vi "Z-Scan-Simulation-Analysis-first-point.vi"() -> ()   [LabVIEW 2014]
doc: "André Romero - 2016\nandretec@ifsc.usp.br"
uses:
  <vilib>/Analysis/baseanly.llb/Mean (DBL).vi
  <vilib>/Utility/file.llb/Write To Spreadsheet File (DBL).vi
  <vilib>/Analysis/NI_AALBase.lvlib
panel:
  out "error (%)":dbl(graph)
  out "Waveform Graph":dbl[][](graph)
  out "Delay VI mean":dbl=63.55555555555556 format="%0.2f"
  out "Delay DAQ mean":dbl=253.55555555555554 format="%0.2f"
  in  "stop":bool
  out "Process time":string="0:00:27"
  out "Array":dbl[](array[numeric])=[2.7399115920461927]
  out "delay (ms)":u32=27328
  in  "milliseconds to wait":u32
  out "mean tf/ti":dbl=2.7399115920461927 format="%0.3f"
  out "status media":i32
  in  "Médias":i32=1 min=1
  out "min value":dbl=2.716291312943804
  out "max value":dbl=2.7530073421259127
  out "Dellay VI":u32(graph)=9
  out "Delay DAQ":u32(graph)=252
  in  "number of samples":i32=40000
  in  "rate":dbl=200000.0 format="%#_13g"
  out "variance":dbl=4.33248215247306e-05 format="%0.6f"
  out "standard deviation":dbl=0.006582159336018128 format="%0.6f"
  out "mean":dbl=2.736901171579517 format="%0.6f"
  out "Delta voltage":dbl=0.03671602918210848 format="%#_8g"
  out "Number of samples":i32=9
  in  "Save ?":bool=TRUE
  in  "delay between points (ms)":u32
  out "Z-Scan Graph":dbl[](graph)=[2.735132708454353, 2.738947350836858, 2.734655244051734, 2.7396822438623687, 2.7278277474129107, 2.7387763962228693, 2.736558085660297, 2.7323997631539765, 2.738221107624196, 2.7393305632862397, 2.741314993759599, 2.747504778022689, 2.738857646673517, 2.730907003892475, 2.732997610548393, 2.7267654500428216, 2.7348215281721826, 2.737937468343614, 2.726070168151901, 2.731887449619976, 2.732414299906183, 2.7330931378202687, 2.716291312943804, 2.7303619340530645, 2.7369114862989874, 2.731523112752885, 2.7354675161048174, 2.7298018305712075, 2.7284991278572837, 2.737353103281323, 2.7327358431598725, 2.734910344261488, 2.7378594937125103, 2.7502146828530214, 2.7337306242369928, 2.739842480175337, 2.7315173269319546, 2.738028284846607, 2.75184747183654, 2.734010133292254, 2.739883879966676, 2.7530073421259127, 2.7364398773661778, 2.7380245402985475, 2.746210731914264, 2.74784258473236, 2.746055600985261, 2.744685689686615, 2.7373947781805184, 2.742865724075715, 2.7398119555480935, 2.7460854422451066, 2.741835143466216, 2.724498522334739, 2.7360680289422383, 2.7324008327222256, 2.7296285024348417, 2.733434961351708, 2.741336308672092, 2.7279657751965862, 2.740709507192904, 2.7400586240991918, 2.739035501835608, 2.7442928765615813, 2.736082802692787, 2.7289248052339135, 2.734834467568928, 2.7227483022204564, 2.73278233554788, 2.732269078647335, 2.7273725581509534, 2.7374985614049385, 2.7403197210099997, 2.7428918309602253, 2.7494572970150637, 2.7288847122884303, 2.7411122138760424, 2.7408703110680195, 2.7347213443213247, 2.7386168772101653, 2.7320536866131246, 2.7323118031594973, 2.7421055815034725, 2.741757853433335, 2.732606885118174, 2.7258367239769905, 2.7501519595100596, 2.737371798824078, 2.731794368257389, 2.7411112883575326, 2.7319720404070353, 2.7423628600299246, 2.7386655586714026, 2.738447831787006, 2.744117336184531, 2.740055256798649, 2.7381788823262183, 2.7463663278142176, 2.7369687172918487, 2.7399115920461927]
  in  "N Points":i32=100
  in  "GO":bool
  out "Z-Scan graph":dbl[][](graph)
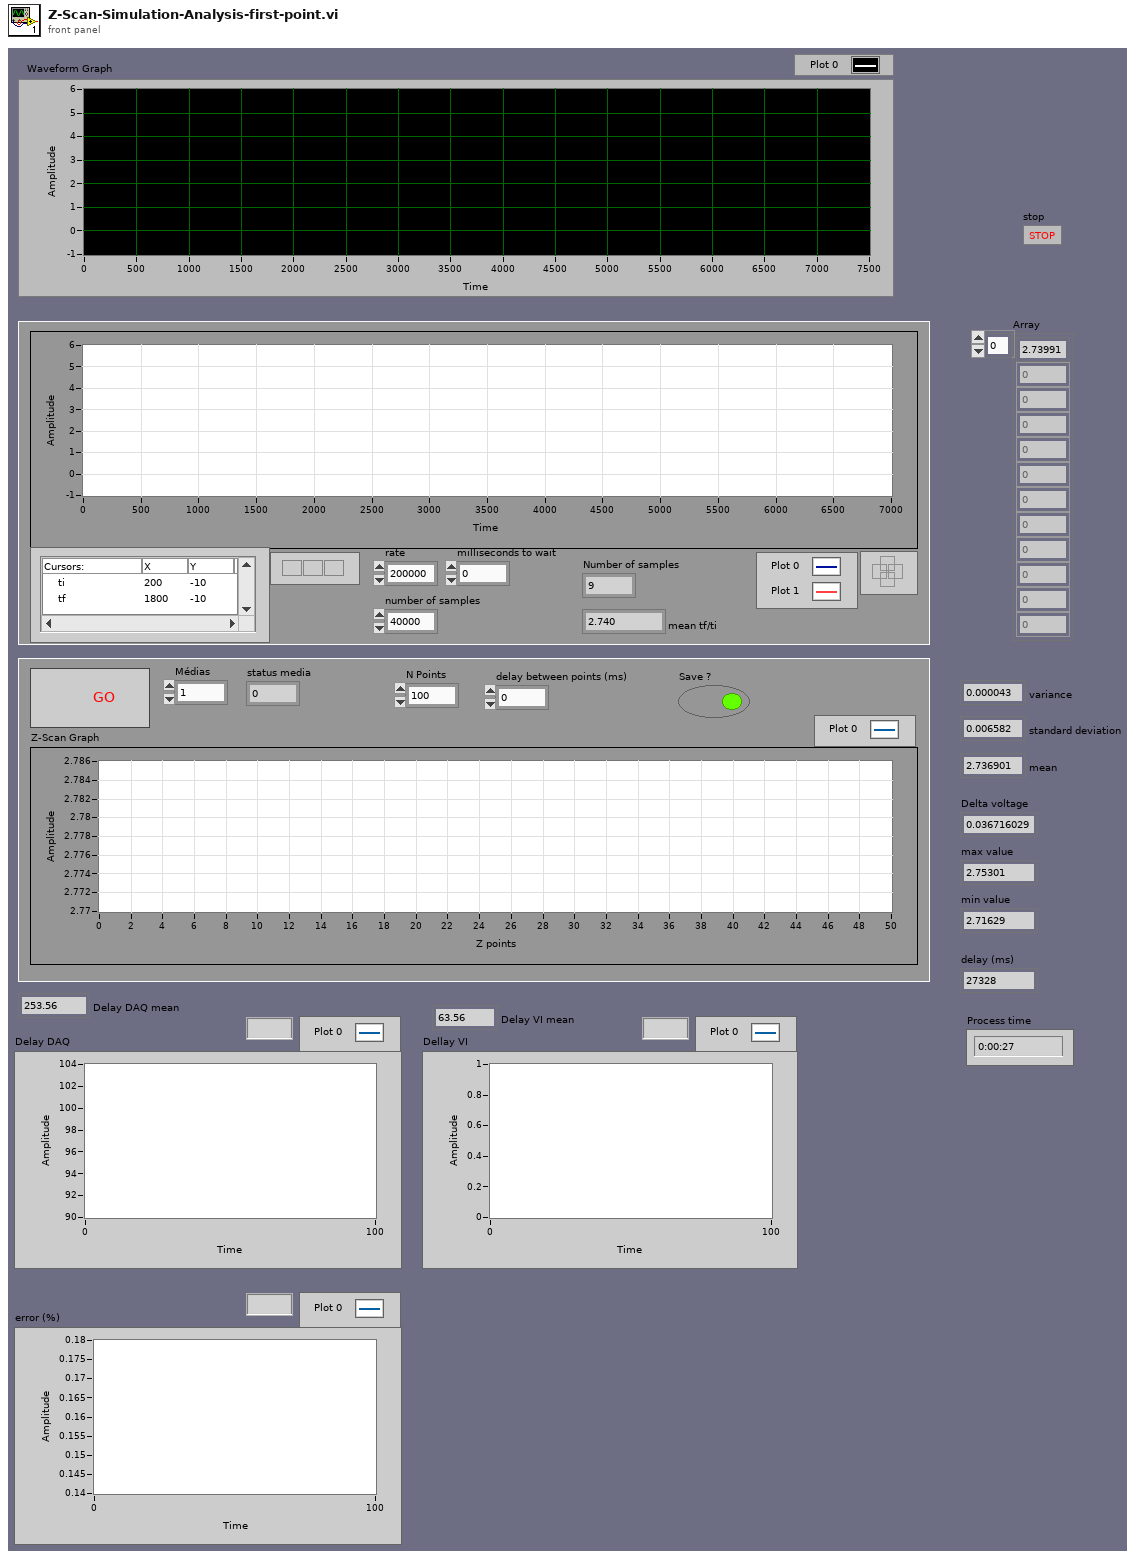
[diagram p1: front panel]
types:
  T1 = typedef "LVCursorListTypeDef.ctl" = cluster{"Name":string, "Color":u32, "Style":u8, "Point Style":u8, "Name Visible":bool, "Allow Drag":bool, "Cursor Mode":u32, "Plot":i32, "Index":i32, "Position":cluster{"X":dbl, "Y":dbl}, "X Scale":u32, "Y Scale":u32, "Watch Plots":i32[], "Watch All Plots":bool, "Plot Area":i32, "Label Offset":cluster{"X":dbl, "Y":dbl}}[]
  T2 = cluster{"Name":string, "Color":u32, "Style":u8, "Point Style":u8, "Name Visible":bool, "Allow Drag":bool, "Cursor Mode":u32, "Plot":i32, "Index":i32, "Position":cluster{"X":dbl, "Y":dbl}, "X Scale":u32, "Y Scale":u32, "Watch Plots":i32[], "Watch All Plots":bool, "Plot Area":i32, "Label Offset":cluster{"X":dbl, "Y":dbl}}
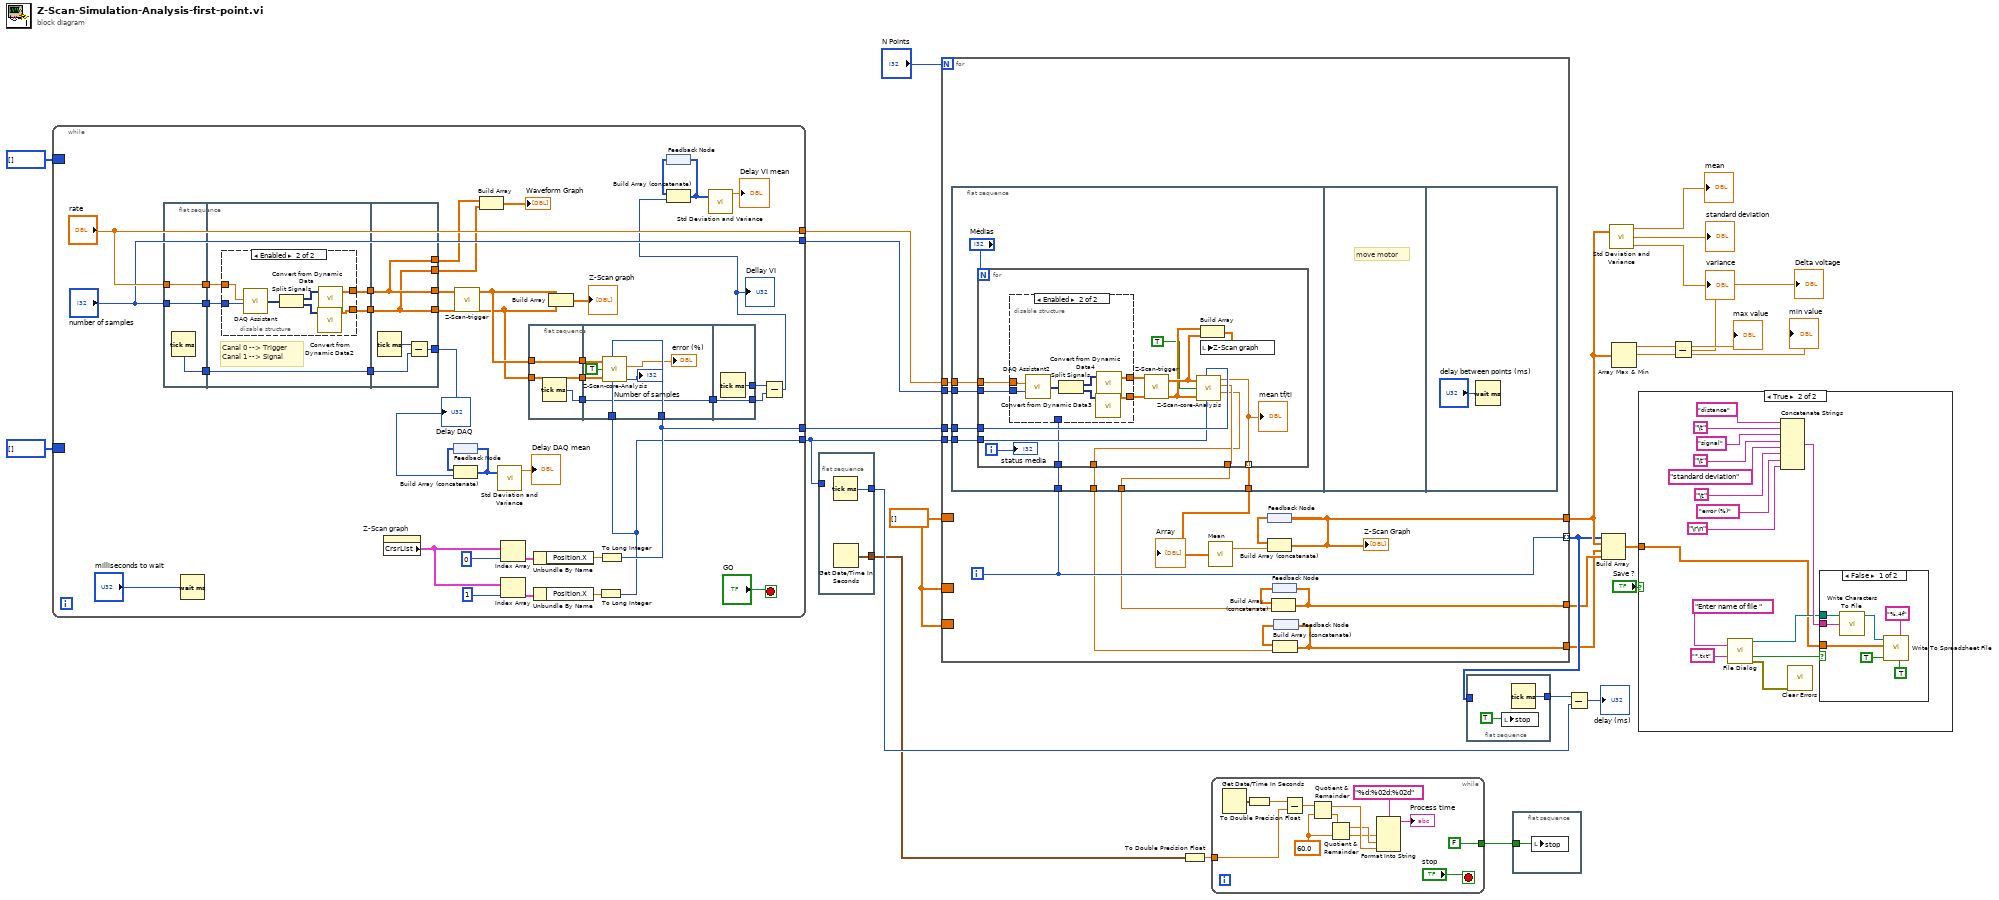
[diagram p0: block diagram]
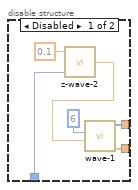
[diagram p2: hidden frame]
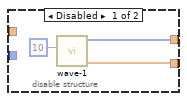
[diagram p3: hidden frame]
diagram:
  w3 = dbl[] []
  n1 = while {
    tunnel: [w58] -> w26
    tunnel: [w57] -> w13
    tunnel: ["rate"] -> w22
    tunnel: ["number of samples"] -> w21
    border: u32[] [] -> [_]
    border: u32[] [] -> [_]
    stop <- "GO" stop-if-true
    n2 = flat-sequence {
      tunnel: "number of samples" -> [w82]
      tunnel: "rate" -> [w83]
      tunnel: [w83] -> w51
      tunnel: [w82] -> w50
      tunnel: [w81] -> w47
      tunnel: w51 -> [w86]
      tunnel: w50 -> [w85]
      tunnel: [w88] -> w49
      tunnel: [w87] -> w48
      tunnel: w47 -> [w84]
      tunnel: [w84] -> w46
      tunnel: [w99] -> w55
      tunnel: [w100] -> w56
      tunnel: w49 -> [w100]
      tunnel: w48 -> [w99]
      tunnel: w46 -> [w102]
      tunnel: [w101] -> w37
      tunnel: [w100] -> w29
      tunnel: [w99] -> w28
      frame #0 {
        n3 = Tick Count (ms)() -> (millisecond timer value=w81:u32)
      }
      frame #1 {
        # "Canal 0 --> Trigger\nCanal 1 --> Signal"
        n4 = disable-structure shown="Enabled" {
          disable-tunnel: [w90 w95] -> w88
          disable-tunnel: [w89 w94] -> w87
          disable-tunnel: w86 -> [_ w98]
          disable-tunnel: w85 -> [_ w97]
          frame Disabled {
            n5 = call "wave-1.vi"("N cycles"=i64 10) -> ("signal"=w89:dbl[], "trigger"=w90:i32[])  [unwired: 7 in]
          }
          frame Enabled {
            n6 = call "DAQ Assistant"("rate"=w98, "number of samples"=w97) -> ("data"=w96:dynamicdata)  [unwired: 15 in, 2 out]
            n7 = Split Signals(w96) -> (w92:dynamicdata, w93:dynamicdata)  [unwired: 2 in]
            n8 = call "Convert from Dynamic Data2"("Dynamic Data Type"=w93) -> ("Array"=w94:dbl[])  [unwired: 3 in]
            n9 = call "Convert from Dynamic Data"("Dynamic Data Type"=w92) -> ("Array"=w95:dbl[])  [unwired: 3 in]
          }
        }
      }
      frame #2 {
        n10 = Tick Count (ms)() -> (millisecond timer value=w103:u32)
        n11 = Subtract(x=w103, y=w102) -> (x-y=w101:u32)
      }
    }
    n12 = Wait (ms)(milliseconds to wait="milliseconds to wait") -> ()  [unwired: 1 out]
    n13 = property on="Z-Scan graph" class="WFGraph (strict)"() -> ("CrsrList"=w66:T1)  [unwired: 2 in, 2 out]
    n14 = feedback #1() -> (w38:u32[])
    n15 = Build Array (concatenate)(w38, w37) -> (w36:u32[])
    n16 = feedback-in #1(w36) -> ()
    n17 = call "Z-Scan-trigger.vi"("signal in"=w55, "trigger in"=w56) -> ("signal out"=w30:dbl[], "trigger out"=w54:dbl[])  [unwired: 5 in, 1 out]
    n18 = Build Array(w29, w28) -> (→"Waveform Graph":dbl[][])
    n19 = call <vilib>:"Std Deviation and Variance.vi"("X"=w36) -> ("mean"=→"Delay DAQ mean":dbl)  [unwired: 1 in, 2 out]
    n20 = Index Array(array=w66, index=0) -> (element=w64:T2)
    n21 = Index Array(array=w66, index=1) -> (element=w63:T2)
    n22 = flat-sequence {
      tunnel: w30 -> [w69]
      tunnel: w54 -> [w70]
      tunnel: [w70] -> w45
      tunnel: [w69] -> w44
      tunnel: [w68] -> w42
      tunnel: w58 -> [w77]
      tunnel: w57 -> [w76]
      tunnel: w45 -> [w75]
      tunnel: w44 -> [w74]
      tunnel: w42 -> [w73]
      tunnel: [w73] -> w41
      tunnel: [w80] -> w43
      tunnel: w41 -> [w79]
      tunnel: [w79] -> w40
      frame #0 {
        n23 = Tick Count (ms)() -> (millisecond timer value=w68:u32)
      }
      frame #1 {
        n24 = call "Z-Scan-core-Analysis.vi"("trigger in"=w75, "ti"=w77, "First point"=TRUE, "signal in"=w74, "tf"=w76) -> ("error (%)"=→"error (%)":dbl, "number of samples"=→"Number of samples":i32)  [unwired: 2 out]
      }
      frame #2 {
        n25 = Tick Count (ms)() -> (millisecond timer value=w80:u32)
      }
    }
    n26 = Unbundle By Name(w64) -> ("Position.X"=w62:dbl)
    n27 = Unbundle By Name(w63) -> ("Position.X"=w61:dbl)
    n28 = Build Array(w30, w54) -> (→"Z-Scan graph":dbl[][])
    n29 = To Long Integer(number=w61) -> (32bit integer=w57:i32)
    n30 = To Long Integer(number=w62) -> (32bit integer=w58:i32)
    n31 = feedback #2() -> (w34:u32[])
    n32 = Subtract(x=w43, y=w40) -> (x-y=w33:u32)
    "Dellay VI" <- w33
    n33 = Build Array (concatenate)(w34, w33) -> (w32:u32[])
    n34 = feedback-in #2(w32) -> ()
    n35 = call <vilib>:"Std Deviation and Variance.vi"("X"=w32) -> ("mean"=→"Delay VI mean":dbl)  [unwired: 1 in, 2 out]
    "Delay DAQ" <- w37
  }
  n36 = flat-sequence {
    tunnel: w13 -> [_]
    tunnel: [w105] -> w10
    tunnel: [w104] -> w7
    frame #0 {
      n37 = Tick Count (ms)() -> (millisecond timer value=w105:u32)
      n38 = Get Date/Time In Seconds() -> (seconds since 1Jan1904=w104:timestamp)
    }
  }
  n39 = for {
    N: "N Points" -> [_]
    tunnel: w26 -> [w120]
    tunnel: w13 -> [w119]
    tunnel: [w117] -> w12 mode=indexing
    border: w3 -> [_]
    tunnel: [w116] -> w14
    tunnel: w22 -> [w115]
    tunnel: w21 -> [w114]
    border: w3 -> [_]
    tunnel: [w109] -> w2
    border: w3 -> [_]
    tunnel: [w106] -> w1
    i -> [w117]
    n40 = flat-sequence {
      tunnel: w120 -> [w129]
      tunnel: w119 -> [w128]
      tunnel: [w127] -> w113
      tunnel: w117 -> [w126]
      tunnel: w115 -> [w125]
      tunnel: w114 -> [w124]
      tunnel: [w122] -> w110
      tunnel: [w121] -> w107
      frame #0 {
        n41 = for {
          N: "Médias" -> [_]
          tunnel: w129 -> [w144]
          tunnel: w128 -> [w143]
          tunnel: [w142] -> w127 mode=indexing
          tunnel: w126 -> [w136]
          tunnel: w125 -> [w135]
          tunnel: w124 -> [w134]
          tunnel: [w131] -> w122
          tunnel: [w130] -> w121
          i -> [w133]
          n42 = disable-structure shown="Enabled" {
            disable-tunnel: [w150 w154] -> w141
            disable-tunnel: [w149 w153] -> w140
            disable-tunnel: w136 -> [w145 _]
            disable-tunnel: w135 -> [_ w152]
            disable-tunnel: w134 -> [_ w151]
            frame Disabled {
              n43 = call "z-wave-2.vi"("index"=w145, "amplitutude"=0.1) -> ("element"=w146:dbl)  [unwired: 1 in, 2 out]
              n44 = call "wave-1.vi"("slope"=w146, "N cycles"=i64 6) -> ("signal"=w149:dbl[], "trigger"=w150:i32[])  [unwired: 6 in]
            }
            frame Enabled {
              n45 = call "DAQ Assistant2"("rate"=w152, "number of samples"=w151) -> ("data"=w155:dynamicdata)  [unwired: 15 in, 2 out]
              n46 = Split Signals(w155) -> (w157:dynamicdata, w156:dynamicdata)  [unwired: 2 in]
              n47 = call "Convert from Dynamic Data3"("Dynamic Data Type"=w156) -> ("Array"=w153:dbl[])  [unwired: 3 in]
              n48 = call "Convert from Dynamic Data4"("Dynamic Data Type"=w157) -> ("Array"=w154:dbl[])  [unwired: 3 in]
            }
          }
          n49 = call "Z-Scan-trigger.vi"("signal in"=w140, "trigger in"=w141) -> ("signal out"=w137:dbl[], "trigger out"=w138:dbl[])  [unwired: 5 in, 1 out]
          n50 = call "Z-Scan-core-Analysis.vi"("trigger in"=w138, "ti"=w144, "First point"=TRUE, "signal in"=w137, "tf"=w143) -> ("mean tf/ti"=w142:dbl, "error (%)"=w131:dbl, "standard deviation"=w130:dbl)  [unwired: 1 out]
          "mean tf/ti" <- w142
          n51 = Build Array(w137, w138) -> (w139:dbl[][])
          n52 = local write "Z-Scan graph"(w139) -> ()
          "status media" <- w133
        }
      }
      frame #1 {
        # "move motor"
      }
      frame #2 {
        n53 = Wait (ms)(milliseconds to wait="delay between points (ms)") -> ()  [unwired: 1 out]
      }
    }
    n54 = call-poly <vilib>:"Mean.vi"("X"=w113) -> ("mean"=w112:dbl)  [unwired: 1 out]
    n55 = feedback #3() -> (w118:dbl[])
    n56 = Build Array (concatenate)(w118, w112) -> (w116:dbl[])
    "Z-Scan Graph" <- w116
    n57 = feedback-in #3(w116) -> ()
    n58 = feedback #4() -> (w111:dbl[])
    n59 = Build Array (concatenate)(w111, w110) -> (w109:dbl[])
    n60 = feedback-in #4(w109) -> ()
    n61 = feedback #5() -> (w108:dbl[])
    n62 = Build Array (concatenate)(w108, w107) -> (w106:dbl[])
    n63 = feedback-in #5(w106) -> ()
    "Array" <- w113
  }
  n64 = To Double Precision Float(number=w7) -> (double precision float=w8:dbl)
  n65 = while {
    tunnel: w8 -> [w164]
    tunnel: [FALSE] -> w6
    stop <- "stop" stop-if-true
    w169 = 60.0 ("y")
    n66 = Get Date/Time In Seconds() -> (seconds since 1Jan1904=w171:timestamp)
    n67 = To Double Precision Float(number=w171) -> (double precision float=w165:dbl)
    n68 = Subtract(x=w165, y=w164) -> (x-y=w163:dbl)
    n69 = Quotient & Remainder(x=w163, y=w169) -> (x-y*floor(x/y)=w168:dbl, floor(x/y)=w170:dbl)
    n70 = Quotient & Remainder(x=w170, y=w169) -> (x-y*floor(x/y)=w167:dbl, floor(x/y)=w166:dbl)
    n71 = Format Into String(format string="%d:%02d:%02d", w166, w167, w168) -> (resulting string=→"Process time":string)  [unwired: 2 in, 1 out]
  }
  n72 = flat-sequence {
    tunnel: w12 -> [_]
    tunnel: [w173] -> w11
    frame #0 {
      n73 = local write "stop"(TRUE) -> ()
      n74 = Tick Count (ms)() -> (millisecond timer value=w173:u32)
    }
  }
  n75 = flat-sequence {
    tunnel: w6 -> [w174]
    frame #0 {
      n76 = local write "stop"(w174) -> ()
    }
  }
  n77 = Subtract(x=w11, y=w10) -> (x-y=→"delay (ms)":u32)
  n78 = Build Array(w12, w14, w1, w2) -> (w24:dbl[][])
  n79 = call <vilib>:"Std Deviation and Variance.vi"("X"=w14) -> ("mean"=→"mean":dbl, "standard deviation"=→"standard deviation":dbl, "variance"=→"variance":dbl)  [unwired: 1 in]
  n80 = Array Max & Min(array=w14) -> (max value=w20:dbl, min value=w19:dbl)  [unwired: 2 out]
  "max value" <- w20
  "min value" <- w19
  n81 = case shown="True" "Save ?" {
    tunnel: w24 -> [_ w182]
    frame False {
    }
    frame True {
      n82 = call "File Dialog"("prompt"="Enter name of file ", "pattern (all files)"="*.txt") -> ("selected path"=w185:path, "cancelled"=w187:bool, "error out"=w186:errorcluster)  [unwired: 10 in, 1 out]
      n83 = Concatenate Strings("distance", "\t", "signal", "\t", "standard deviation", "\t", "error (%)", "\r\n") -> (w189:string)
      n84 = call <vilib>:"Clear Errors.vi"("error in (no error)"=w186) -> ()  [unwired: 5 in, 2 out]
      n85 = case shown="False" w187 {
        tunnel: w185 -> [w196 _]
        tunnel: w182 -> [w193 _]
        tunnel: w189 -> [w192 _]
        frame False {
          n86 = call <vilib>:"Write Characters To File.vi"("character string"=w192, "file path (dialog if empty)"=w196) -> ("new file path (Not A Path if cancelled)"=w195:path)  [unwired: 3 in]
          n87 = call-poly <vilib>:"Write To Spreadsheet File.vi"("transpose? (no:F)"=TRUE, "format (%.3f)"="%.4f", "append to file? (new file:F)"=TRUE, "2D data"=w193, "file path (dialog if empty)"=w195) -> ()  [unwired: 3 in, 1 out]
        }
        frame True {
        }
      }
    }
  }
  n88 = Subtract(x=w20, y=w19) -> (x-y=→"Delta voltage":dbl)
